vi "Configure Channel.vi"(8 "error in (no error)":errorcluster, 10 "DAQmx Task In":refnum<k21>, 11 "BridgeChannel in":refnum<class "BridgeChannel.lvclass">) -> (0 "error out":errorcluster, 2 "DAQmx Task":refnum<k21>)   [LabVIEW 2023, in "VolatusDAQConfig.lvlib" / "BridgeChannel.lvclass"]
uses:
  BridgeChannel.lvclass
  VolatusConfig/VolatusConfigElement/VolatusConfigElement.lvclass/VolatusConfigElement.ctl
  BridgeChannel.lvclass/BridgeChannel.ctl
  VolatusConfig/VolatusConfigElement/Element.vi
  VolatusConfig/VolatusConfigElement/Lookup Child by Name.vi
  VolatusConfig/Channel/Channel Config.lvclass
  lv-cdm/CDM-Config/Config Element/Lookup Child by Name.vi
  lv-cdm/CDM-Config/Config Element/Value (String).vi
  <vilib>/DAQmx/create/channels.llb/DAQmx Create Channel (AI-Bridge).vi
  VolatusConfig/VolatusConfigElement/VolatusConfigElement.lvclass
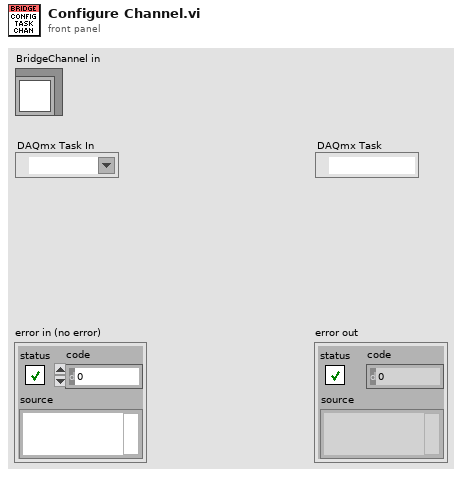
[diagram p1: front panel]
types:
  T1 = cluster{"bridge configuration":i32, "voltage excitation source":i32, "voltage excitation value":dbl, "nominal bridge resistance":dbl}
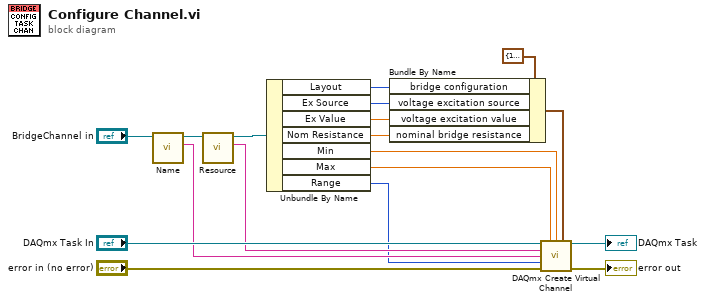
[diagram p0: block diagram]
diagram:
  n1 = call "Name.vi"("VolatusConfigElement in"="BridgeChannel in") -> ("Name"=w3:string, "VolatusConfigElement out"=w6:refnum<class "BridgeChannel.lvclass">)  [unwired: 8 in, 1 out]
  n2 = call "Resource.vi"("Channel in"=w6) -> ("Resource"=w2:string, "Channel out"=w5:refnum<class "BridgeChannel.lvclass">)  [unwired: 8 in, 1 out]
  n3 = Unbundle By Name(w5) -> ("Layout"=w12:i32, "Ex Source"=w11:i32, "Ex Value"=w10:dbl, "Nom Resistance"=w9:dbl, "Min"=w8:dbl, "Max"=w7:dbl, "Range"=w1:i32)
  n4 = Bundle By Name(cluster=T1 {"bridge configuration"=10182, "voltage excitation source"=10200, "voltage excitation value"=2.5, "nominal bridge resistance"=350.0} ("bridge information"), "bridge configuration"=w12, "voltage excitation source"=w11, "voltage excitation value"=w10, "nominal bridge resistance"=w9) -> (w13:T1)
  n5 = call-poly <vilib>:"DAQmx Create Virtual Channel.vi"("task in"="DAQmx Task In", "maximum value"=w7, "minimum value"=w8, "bridge information"=w13, "physical channels"=w2, "name to assign"=w3, "units"=w1, "error in"="error in (no error)") -> ("task out"=→"DAQmx Task":refnum<k21>, "error out"=→"error out":errorcluster)  [unwired: 6 in]
